vi "Callback - Get Plottable Names.vi"(8 "error in (no error)":errorcluster, 11 "BluePlotHandle in":refnum<class "BluePlotHandle.lvclass">) -> (0 "error out":errorcluster, 2 "Plottable Names":string[](array[string]), 3 "BluePlotHandle out":refnum<class "BluePlotHandle.lvclass">)   [LabVIEW 2021, in "BluePlot.lvlib" / "BluePlotHandle.lvclass"]
uses:
  BluePlotHandle.lvclass
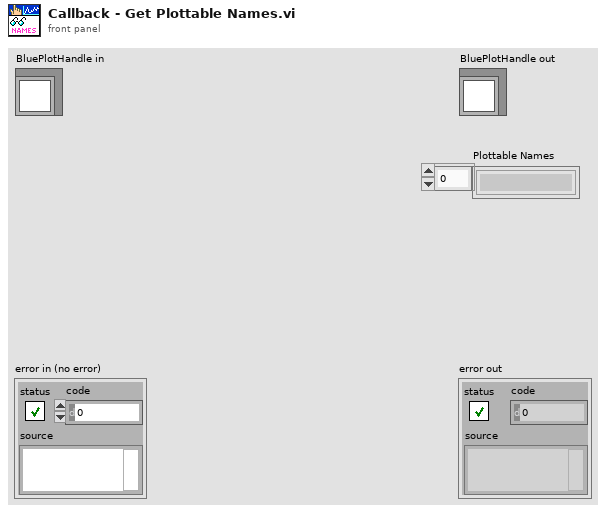
[diagram p1: front panel]
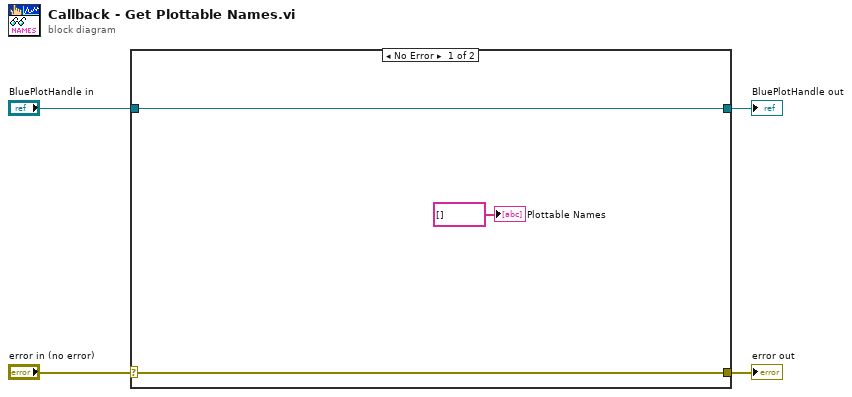
[diagram p0: block diagram]
diagram:
  n1 = case shown="No Error" "error in (no error)" {
    selector: "error in (no error)" -> [w6 w9]
    tunnel: [w6 w9] -> w3
    tunnel: [w7 w8] -> w1
    tunnel: "BluePlotHandle in" -> [w7 w8]
    frame No Error {
      "Plottable Names" <- string[] [] ("Names")
    }
    frame Error {
    }
  }
  "error out" <- w3
  "BluePlotHandle out" <- w1
